vi "Test Read HDI Fiducials.vi"() -> ()   [LabVIEW 2011]
uses:
  CameraTool Class.lvclass
  Gantry Class/Gantry Class.lvclass
panel:
  in  "Config Folder":path=path "C:/Users/Husker/Desktop/gantry/Config"
  in  "HOME?":bool=TRUE
  out "Error":errorcluster
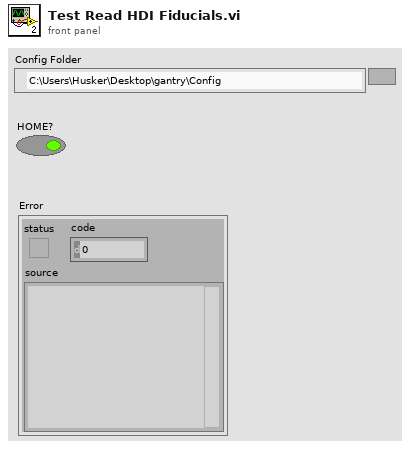
[diagram p1: front panel]
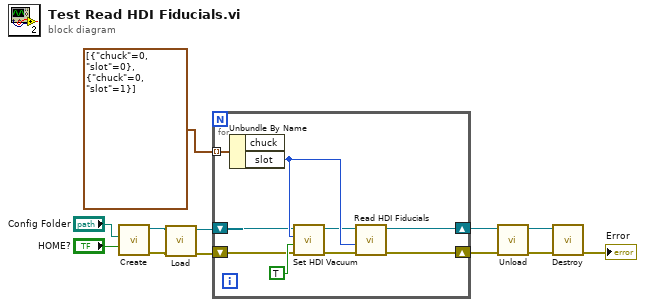
[diagram p0: block diagram]
diagram:
  n1 = call "Create.vi"("HOME?"="HOME?", "Config Folder"="Config Folder") -> ("error out"=w9:errorcluster, "Gantry out"=w10:refnum<class "Gantry Class.lvclass">)  [unwired: 8 in]
  n2 = call "Load.vi"("error in (no error)"=w9, "Gantry In"=w10) -> ("error out"=w1:errorcluster, "CameraTool out"=w2:refnum<class "CameraTool Class.lvclass">)  [unwired: 8 in]
  n3 = for {
    shift-right: [w20] -> w5
    shift-left: w2 -> [w14]
    tunnel: cluster{"chuck":u32, "slot":u32}[] [{"chuck"=0, "slot"=0}, {"chuck"=0, "slot"=1}] -> [w21] mode=indexing
    shift-right: [w19] -> w6
    shift-left: w1 -> [w16]
    n4 = Unbundle By Name(w21) -> ("slot"=w18:u32)  [unwired: 1 out]
    n5 = call "Set HDI Vacuum.vi"("error in"=w16, "On/Off"=TRUE, "Slot Number"=w18, "Gantry in"=w14) -> ("error out"=w15:errorcluster, "Gantry out"=w13:refnum<class "CameraTool Class.lvclass">)  [unwired: 6 in]
    n6 = call-dynamic "Read HDI Fiducials.vi"("error in"=w15, "Slot"=w18, "CameraTool in"=w13) -> ("error out"=w19:errorcluster, "CameraTool out"=w20:refnum<class "CameraTool Class.lvclass">)  [unwired: 7 in]
  }
  n7 = call "Unload.vi"("error in (no error)"=w6, "CameraTool in"=w5) -> ("error out"=w8:errorcluster, "Gantry out"=w7:refnum<class "Gantry Class.lvclass">)  [unwired: 8 in]
  n8 = call "Destroy.vi"("error in"=w8, "Gantry Class in"=w7) -> ("error out"=→"Error":errorcluster)  [unwired: 9 in]
